vi "C8855-01_MakingGate.vi"(8 "MainD":T1 {"G_DIM" format="%.5f"}, 11 "GStep":dbl format="%#.6f") -> (3 "StepGate":i32)   [LabVIEW 2017]
uses:
  C8855_MainD.ctl
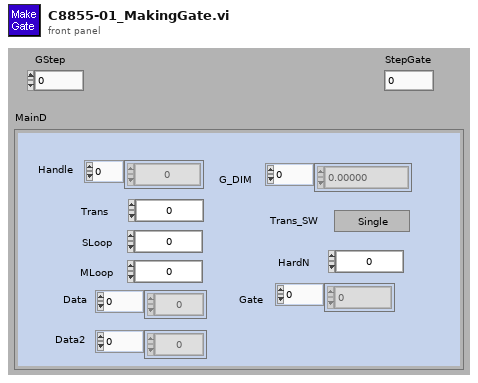
[diagram p1: front panel]
types:
  T1 = typedef "C8855_MainD.ctl" = cluster{"Handle":i64[], "G_DIM":dbl[], "Trans":u16, "Trans_SW":bool, "HardN":i32, "Gate":u8[], "Data":u32[], "Data2":u32[], "SLoop":i32, "MLoop":i32}
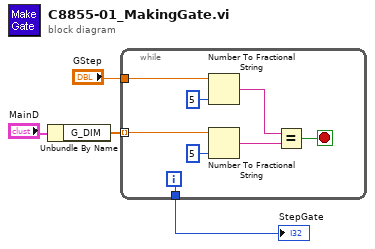
[diagram p0: block diagram]
diagram:
  n1 = Unbundle By Name("MainD") -> ("G_DIM"=w3:dbl[])
  n2 = while {
    tunnel: w3 -> [w7] mode=indexing
    tunnel: "GStep" -> [w8]
    tunnel: [w11] -> w1
    i -> [w11]
    stop <- w12 stop-if-true
    n3 = Number To Fractional String(number=w8, precision (6)=i16 5 ("¸x(6)")) -> (F-format string=w5:string)  [unwired: 2 out]
    n4 = Number To Fractional String(number=w7, precision (6)=i16 5 ("¸x(6)")) -> (F-format string=w6:string)  [unwired: 2 out]
    n5 = Equal?(x=w5, y=w6) -> (x = y?=w12:bool)
  }
  "StepGate" <- w1
